vi "MesurementLoop.vi"(1 "Trav Command":T1 items=["Set Reference", "Read Position", "Move", "StopMotors"]) -> ()   [LabVIEW 2017]
uses:
  TypeDefs/Position-Info-TD.ctl
  TypeDefs/Trav-Command-TD.ctl
  Controls/saveDataOption.ctl
  Settings/Traverse-Settings-Global.vi
panel:
  out "current time Start":timestamp
  out "current time End":timestamp
  out "Current Iteration":i32
  out "Total No of Iterations":i32
  out "array":dbl[][](array[numeric])
  in  "Position Info IN":T2
  out "Position Info OUT":T2
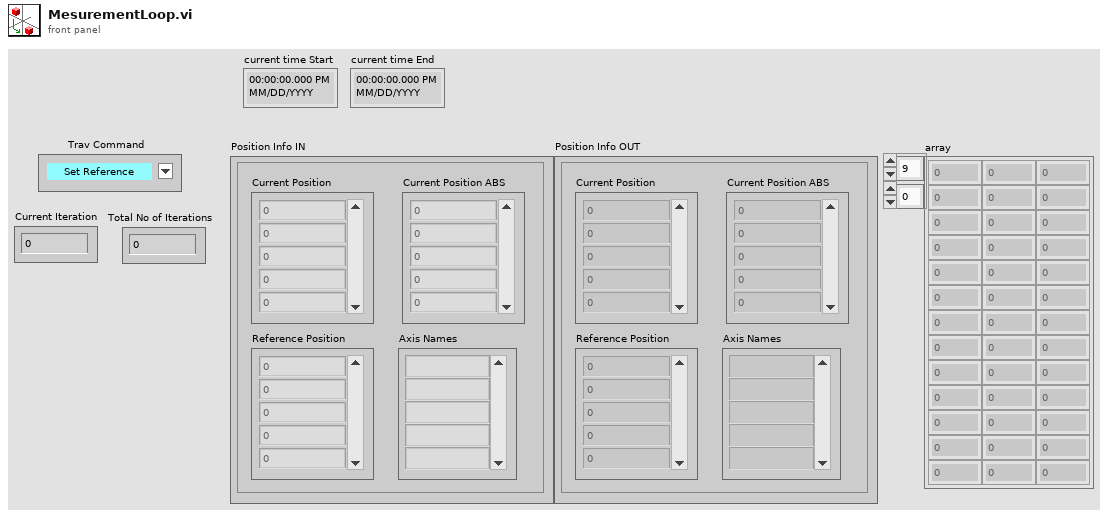
[diagram p1: front panel]
types:
  T1 = typedef "Trav-Command-TD.ctl" = u16
  T2 = typedef "Position-Info-TD.ctl" = cluster{"Current Position ABS":dbl[], "Current Position":dbl[], "Reference Position":dbl[], "Axis Names":string[]}
  T3 = typedef "saveDataOption.ctl" = enum16{"Save Data", "Do Not Save Data"}
  T4 = enum16{"New Measurement", "Post-process Raw Data"}
  T5 = typedef "Settings-Control.ctl" = cluster{"Acceleration":dbl[], "Deceleration":dbl[], "Max Velocity":dbl[], "Speed":dbl, "Pulse/Degree":dbl, "Degre Factor":dbl[], "mm/rotation":dbl[], "Traverse Name":string}
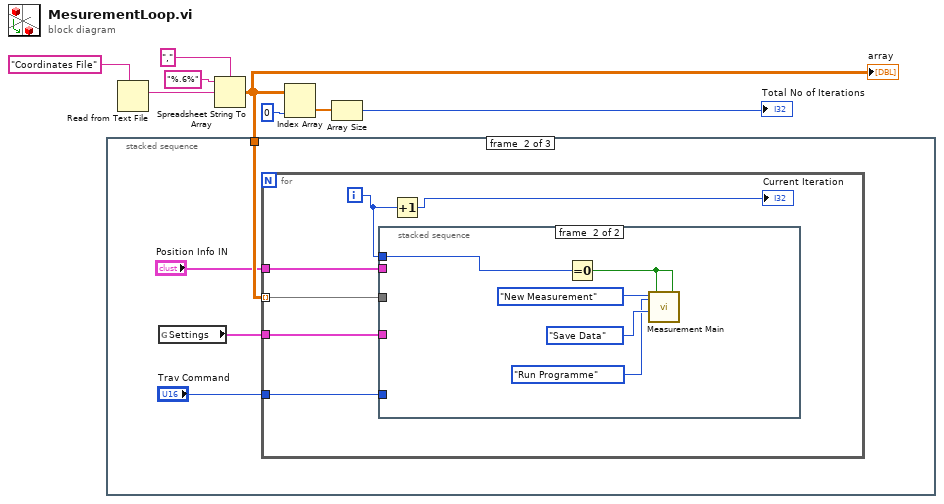
[diagram p0: block diagram]
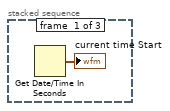
[diagram p2: hidden frame]
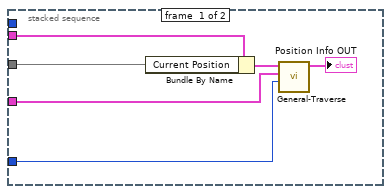
[diagram p3: hidden frame]
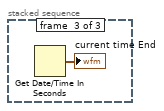
[diagram p4: hidden frame]
diagram:
  n1 = Read from Text File(prompt (Open existing file)="Coordinates File") -> (text=w7:string)  [unwired: 3 in, 3 out]
  n2 = Spreadsheet String To Array(delimiter (Tab)=",", format string="%.6%", spreadsheet string=w7) -> (array=w1:dbl[][])  [unwired: 1 in]
  "array" <- w1
  n3 = stacked-sequence {
    tunnel: w1 -> [_ w13 _]
    frame #0 {
      n4 = Get Date/Time In Seconds() -> (seconds since 1Jan1904=→"current time Start":timestamp)
    }
    frame #1 {
      n5 = global read "Traverse-Settings-Global.vi" "Settings"() -> (w12:T5)
      n6 = for {
        tunnel: w13 -> [w19] mode=indexing
        tunnel: w12 -> [w16]
        tunnel: "Position Info IN" -> [w15]
        tunnel: "Trav Command" -> [w14]
        i -> [w17]
        n7 = stacked-sequence {
          tunnel: w19 -> [w25 _]
          tunnel: w17 -> [_ w30]
          tunnel: w16 -> [w24 _]
          tunnel: w15 -> [w23 _]
          tunnel: w14 -> [w22 _]
          frame #0 {
            n8 = Bundle By Name(cluster=w23, "Current Position"=w25) -> (w21:T2)
            n9 = call "General-Traverse.vi"("Trav Command"=w22, "Settings"=w24, "Position Info IN"=w21) -> ("Position Info OUT"=→"Position Info OUT":T2)  [unwired: 7 in, 1 out]
          }
          frame #1 {
            n10 = Equal To 0?(x=w30) -> (x = 0?=w26:bool)
            n11 = call "Measurement Main.vi"("New Data Post-Pro Folder"=w26, "Setup"=enum16{"Run Programme", "Show Setup"}."Run Programme", "Save Data Option"=saveDataOption."Save Data", "New Measurement Folder"=w26, "Data Acquisition"=T4."New Measurement") -> ()  [unwired: 1 in]
          }
        }
        n12 = Increment(x=w17) -> (x+1=→"Current Iteration":i32)
      }
    }
    frame #2 {
      n13 = Get Date/Time In Seconds() -> (seconds since 1Jan1904=→"current time End":timestamp)
    }
  }
  n14 = Index Array(array=w1, index (col)=0 ("disabled index (col)")) -> (element=w3:dbl[])  [unwired: 1 in]
  n15 = Array Size(array=w3) -> (size(s)=→"Total No of Iterations":i32)
